vi "test UUID.vi"() -> ()   [LabVIEW 2014]
uses:
  user.lib/_NEVSTOP/Communicable State Machine(CSM)/Communicable State Machine.lvlib
panel:
  out "Numeric":i32
  out "x != 0?":bool
  out "Array":string[](array[string])
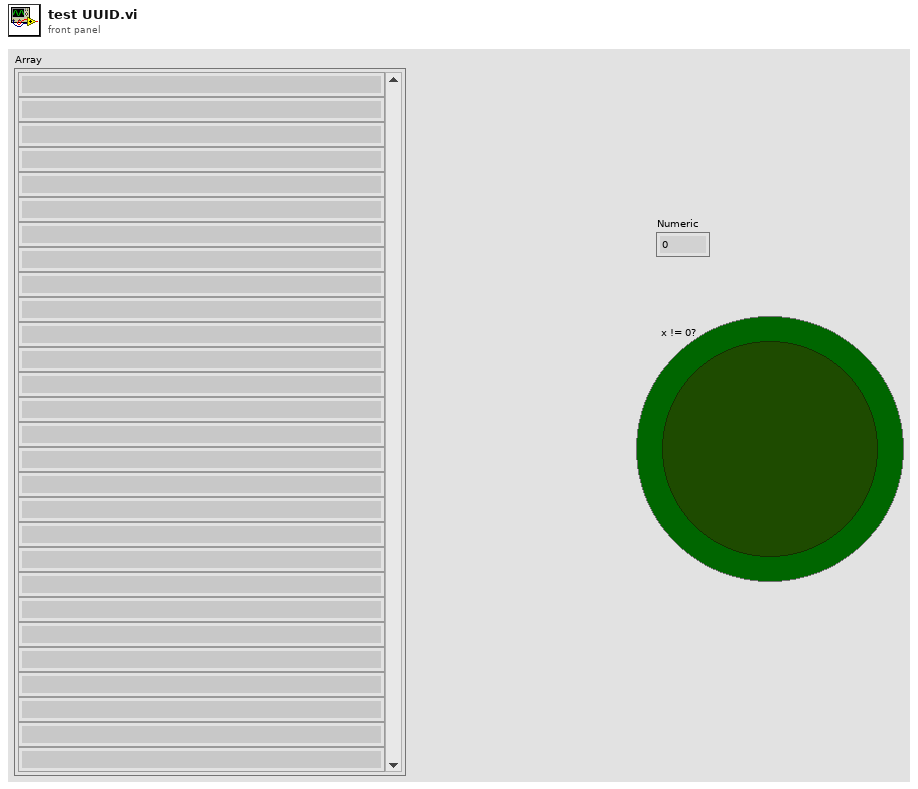
[diagram p1: front panel]
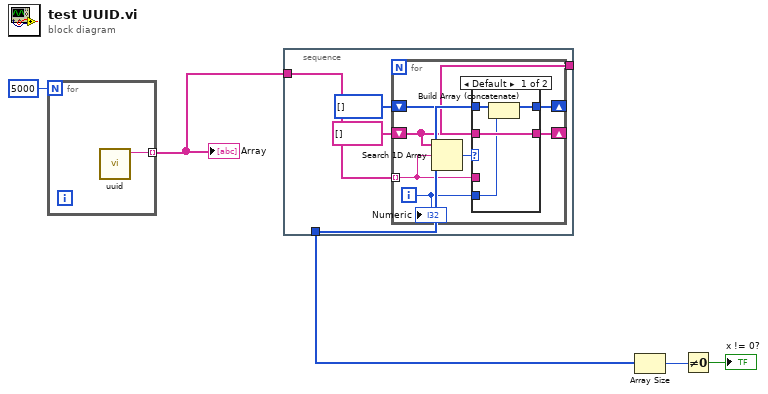
[diagram p0: block diagram]
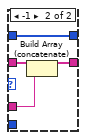
[diagram p2: hidden frame]
diagram:
  n1 = for {
    N: 5000 -> [_]
    tunnel: [w6] -> w4 mode=indexing
    n2 = call "uuid.vi"() -> ("UUID"=w6:string)  [unwired: 11 in]
  }
  "Array" <- w4
  n3 = stacked-sequence {
    tunnel: w4 -> [w7]
    tunnel: [w9] -> _
    tunnel: [w11] -> w3
    frame #0 {
      n4 = for {
        tunnel: w7 -> [w17] mode=indexing
        shift-right: [w16] -> w9
        shift-left: string[] [] -> [w15]
        shift-right: [w13] -> w11
        shift-left: i32[] [] -> [w12]
        i -> [w14]
        n5 = Search 1D Array(1D array=w15, element=w17) -> (index of element=w18:i32)  [unwired: 1 in]
        n6 = case shown="Default" w18 {
          tunnel: w17 -> [_ w26]
          tunnel: [w22 w24] -> w16
          tunnel: w15 -> [w22 w25]
          tunnel: w14 -> [w19 _]
          tunnel: [w20 w23] -> w13
          tunnel: w12 -> [w21 w23]
          frame Default {
            n7 = Build Array (concatenate)(w21, w19) -> (w20:i32[])
          }
          frame -1 {
            n8 = Build Array (concatenate)(w25, w26) -> (w24:string[])
          }
        }
        "Numeric" <- w14
      }
    }
  }
  n9 = Array Size(array=w3) -> (size(s)=w2:i32)
  n10 = Not Equal To 0?(x=w2) -> (x != 0?=→"x != 0?":bool)
